vi "GetDirectionOfSnakePart.vi"(8 "error in (no error)":errorcluster, 11 "tile in":T2) -> (0 "error out":errorcluster, 2 "Stop":bool, 3 "Direction":T1)   [LabVIEW 2020]
doc: "Translates body part tile to a direction it's facing.\nIf head returns Stop=True\nThrows an error if not a body part."
uses:
  TypeDef/tiles-key-trunct.ctl
  TypeDef/direction.ctl
  <vilib>/Utility/error.llb/Error Cluster From Error Code.vi
  <vilib>/ErrorRing/Error Ring.xnode
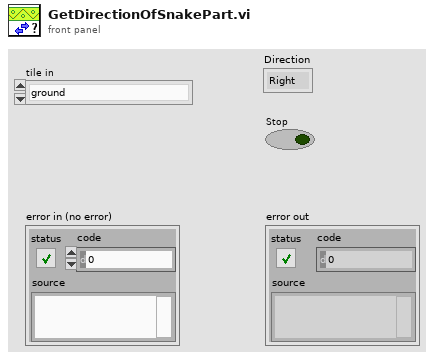
[diagram p1: front panel]
types:
  T1 = typedef "direction.ctl" = enum16{"Right", "Up", "Left", "Down"}
  T2 = typedef "tiles-key-trunct.ctl" = enum16{"ground", "wall", "head (right)", "head (up)", "head (left)", "head (down)", "L-turn (right-up)", "L-turn (up-left)", "L-turn (left-down)", "L-turn (down-right)", "body (right)", "body (up)", "body (left)", "body (down)", "R-turn (right-down)", "R-turn (up-right)", "R-turn (left-up)", "R-turn (down-left)", "tail (right)", "tail (up)", "tail (left)", "tail (down)"}
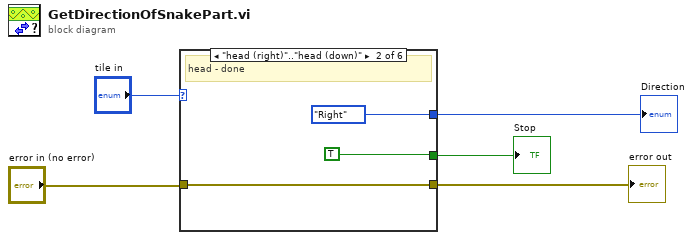
[diagram p0: block diagram]
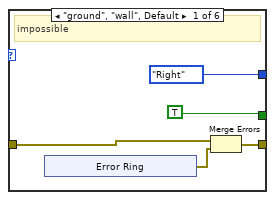
[diagram p2: hidden frame]
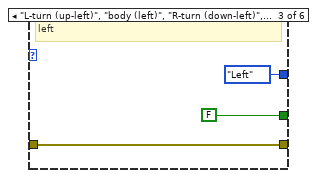
[diagram p3: hidden frame]
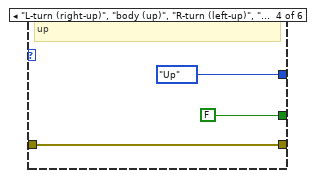
[diagram p4: hidden frame]
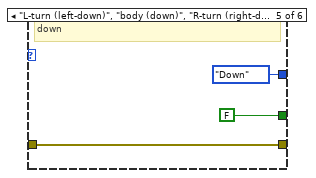
[diagram p5: hidden frame]
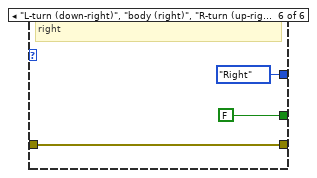
[diagram p6: hidden frame]
diagram:
  n1 = case shown="\"head (right)\"..\"head (down)\"" "tile in" {
    tunnel: [TRUE TRUE FALSE FALSE FALSE FALSE] -> w2
    tunnel: "error in (no error)" -> [w6 w17 w20 w24 w26 w29]
    tunnel: [w7 w17 w20 w24 w26 w29] -> w4
    tunnel: [direction."Right" ("Direction") direction."Right" ("Direction") direction."Left" ("Direction") direction."Up" ("Direction") direction."Down" ("Direction") direction."Right" ("Direction")] -> w5
    frame "ground", "wall", Default {
      # "impossible"
      n2 = xnode "Error Ring"() -> ("error out"=w9:errorcluster)
      n3 = Merge Errors(w6, w9) -> (w7:errorcluster)
    }
    frame "head (right)".."head (down)" {
      # "head - done"
    }
    frame "L-turn (up-left)", "body (left)", "R-turn (down-left)", "tail (left)" {
      # "left"
    }
    frame "L-turn (right-up)", "body (up)", "R-turn (left-up)", "tail (up)" {
      # "up"
    }
    frame "L-turn (left-down)", "body (down)", "R-turn (right-down)", "tail (down)" {
      # "down"
    }
    frame "L-turn (down-right)", "body (right)", "R-turn (up-right)", "tail (right)" {
      # "right"
    }
  }
  "Direction" <- w5
  "error out" <- w4
  "Stop" <- w2
